vi "Check Cal Dates.vi"(11 "Calibration List":T1(array[cluster])) -> (2 "Status":string[](array[string]), 3 "Calibration Status":bool)   [LabVIEW 2010]
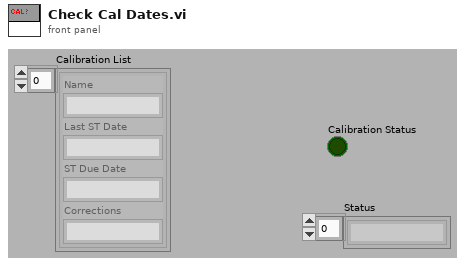
[diagram p1: front panel]
types:
  T1 = cluster{"Name":string, "Last ST Date":string, "ST Due Date":string, "Corrections":string}[]
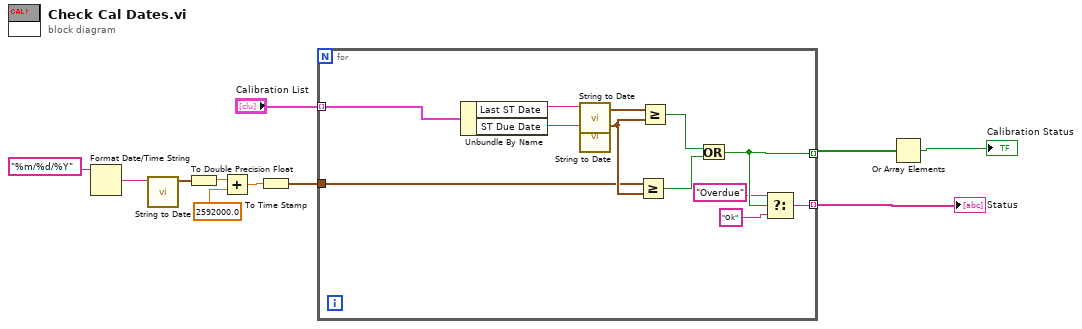
[diagram p0: block diagram]
diagram:
  n1 = Format Date/Time String(time format string (%c)="%m/%d/%Y") -> (date/time string=w2:string)  [unwired: 2 in]
  n2 = call "String to Date.vi"("Cal Due Date"=w2) -> ("time stamp"=w8:timestamp)  [unwired: 10 in]
  n3 = To Double Precision Float(number=w8) -> (double precision float=w7:dbl)
  n4 = Add(x=w7, y=2592000.0) -> (x+y=w5:dbl)
  n5 = To Time Stamp(1:w5) -> (0:w4:timestamp)
  n6 = for {
    tunnel: [w15] -> w11 mode=indexing
    tunnel: "Calibration List" -> [w17] mode=indexing
    tunnel: w4 -> [w16]
    tunnel: [w12] -> w1 mode=indexing
    n7 = Unbundle By Name(w17) -> ("Last ST Date"=w23:string, "ST Due Date"=w22:string)
    n8 = call "String to Date.vi"("Cal Due Date"=w23) -> ("time stamp"=w21:timestamp)  [unwired: 10 in]
    n9 = call "String to Date.vi"("Cal Due Date"=w22) -> ("time stamp"=w20:timestamp)  [unwired: 10 in]
    n10 = Greater Or Equal?(x=w16, y=w20) -> (x >= y?=w19:bool)
    n11 = Greater Or Equal?(x=w21, y=w20) -> (x >= y?=w18:bool)
    n12 = Or(x=w18, y=w19) -> (x .or. y?=w15:bool)
    n13 = Select(t="Overdue", s=w15, f="Ok") -> (s? t:f=w12:string)
  }
  "Status" <- w1
  n14 = Or Array Elements(Boolean array=w11) -> (logical OR=→"Calibration Status":bool)
